vi "Every Value.vi"(8 "error in (no error)":errorcluster, 11 "prefix":string="DEV:") -> (0 "error out":errorcluster, 3 "values":map{string, refnum<class "NT Base.lvclass">}(c390))   [LabVIEW 2020]
uses:
  source/PV Data/NT Base/NT Base.lvclass
  source/PV Data/NT Scalar (Numeric)/NT Scalar (Numeric).lvclass
  C:/Users/eyw68381/source/repos/pvaccess-labview/labview/source/PV Data/NT Scalar/NT Scalar.lvclass
  C:/Users/eyw68381/source/repos/pvaccess-labview/labview/source/PV Data/NT Base/NT Base.lvclass
  source/PV Data/NT Scalar/NT Scalar.lvclass
  source/PV Data/Type Code.ctl
  source/PV Data/PV Data.lvlib
  Every Type Code.ctl
  d16f01a4-6b33-4dc9-a2fb-bc06e15f7701.vi
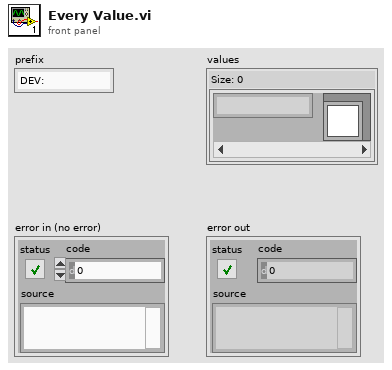
[diagram p1: front panel]
types:
  T1 = typedef "Every Type Code.ctl" = T2[]
  T2 = typedef "PV Access.lvlib/PV Data.lvlib/Type Code.ctl" = enum8{"Null", "Bool", "BoolA", "Int8", "Int8A", "Int16", "Int16A", "Int32", "Int32A", "Int64", "Int64A", "UInt8", "UInt8A", "UInt16", "UInt16A", "UInt32", "UInt32A", "UInt64", "UInt64A", "Float32", "Float32A", "Float64", "Float64A", "String", "StringA", "Struct", "StructA", "Union", "UnionA", "Any", "AnyA"}
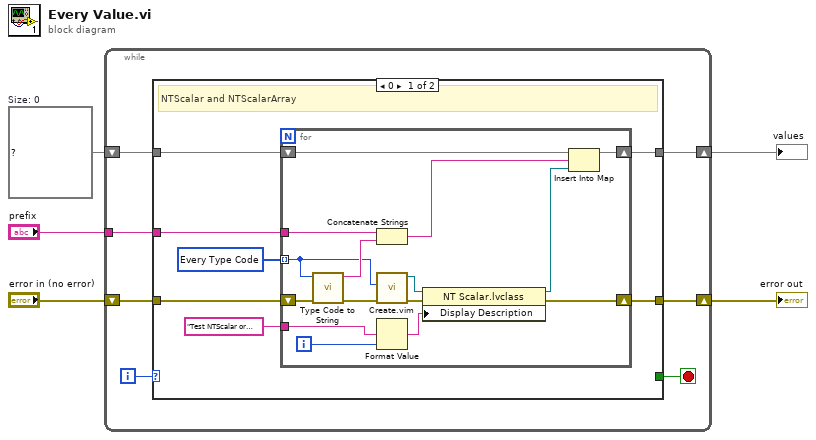
[diagram p0: block diagram]
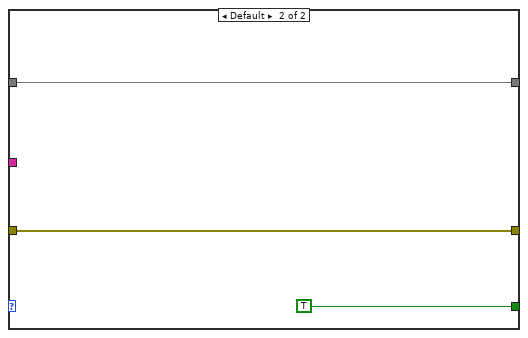
[diagram p2: hidden frame]
diagram:
  w3 = map{string, refnum<class "NT Base.lvclass">} {}  # Size: 0
  n1 = while {
    shift-right: [w11] -> w4
    shift-left: "error in (no error)" -> [w12]
    shift-right: [w9] -> w2
    shift-left: w3 -> [w10]
    tunnel: "prefix" -> [w6]
    i -> [w8]
    stop <- w7 stop-if-true
    n2 = case shown="0" w8 {
      tunnel: w12 -> [w19 w37]
      tunnel: [w18 w37] -> w11
      tunnel: w10 -> [w17 w36]
      tunnel: [w16 w36] -> w9
      tunnel: [_ TRUE] -> w7
      tunnel: w6 -> [w14 _]
      frame 0 {
        w15 = T1 [enum."Bool", enum."Int8", enum."Int16", enum."Int32", enum."Int64", enum."UInt8", enum."UInt16", enum."UInt32", enum."UInt64", enum."Float32", enum."Float64", enum."String", enum."BoolA", enum."Int8A", enum."Int16A", enum."Int32A", enum."Int64A", enum."UInt8A", enum."UInt16A", enum."UInt32A", enum."UInt64A", enum."Float32A", enum."Float64A", enum."StringA"] items=["Null", "Bool", "BoolA", "Int8", "Int8A", "Int16", "Int16A", "Int32", "Int32A", "Int64", "Int64A", "UInt8", "UInt8A", "UInt16", "UInt16A", "UInt32", "UInt32A", "UInt64", "UInt64A", "Float32", "Float32A", "Float64", "Float64A", "String", "StringA", "Struct", "StructA", "Union", "UnionA", "Any", "AnyA"] ("Array")
        # "NTScalar and NTScalarArray"
        n3 = for {
          shift-right: [w29] -> w18
          shift-left: w19 -> [w34]
          shift-right: [w31] -> w16
          shift-left: w17 -> [w32]
          tunnel: w15 -> [w24] mode=indexing
          tunnel: w14 -> [w23]
          tunnel: "Test NTScalar or NTScalarArray PV %d" ("Description") -> [w20]
          i -> [w21]
          n4 = call "Type Code to String.vi"("error in (no error)"=w34, "type code"=w24) -> ("error out"=w33:errorcluster, "string"=w26:string)  [unwired: 8 in]
          n5 = Concatenate Strings(w23, w26) -> (w25:string)
          n6 = call "Create.vim"("error in (no error)"=w33, "initial value"=w24) -> ("error out"=w30:errorcluster, "NT Base out"=w28:refnum<class "NT Scalar.lvclass">)  [unwired: 6 in, 2 out]
          n7 = Format Value(format string=w20, value (0)=w21) -> (output string=w22:string)  [unwired: 1 in]
          n8 = property class="NT Scalar.lvclass"(reference=w28, error in=w30, "Display Description"=w22) -> (reference out=w27:refnum<class "NT Scalar.lvclass">, error out=w29:errorcluster)
          n9 = Insert Into Map(map in=w32, key=w25, value=w27) -> (map out=w31:map{string, refnum<class "NT Base.lvclass">})  [unwired: 2 out]
        }
      }
      frame Default {
      }
    }
  }
  "error out" <- w4
  "values" <- w2
